vi "BonOMM-SAOMM.Test.vi"() -> ()   [LabVIEW 2011] (continued)
                        n5497 = property on="ModifRotation" class="Bool (strict)"("Blinking"=w3909) -> ()  [unwired: 2 in, 2 out]
                        n5498 = property on="ModifDome" class="Bool (strict)"("Blinking"=w3909) -> ()  [unwired: 2 in, 2 out]
                        n5499 = property on="Zénith" class="Bool (strict)"("Blinking"=w3909) -> ()  [unwired: 2 in, 2 out]
                        n5500 = property on="Range" class="Bool (strict)"("Blinking"=w3909) -> ()  [unwired: 2 in, 2 out]
                        n5501 = property on="Écran" class="Bool (strict)"("Blinking"=w3909) -> ()  [unwired: 2 in, 2 out]
                        n5502 = property on="ModifFoyer" class="Bool (strict)"("Blinking"=w3909) -> ()  [unwired: 2 in, 2 out]
                      }
                      frame #1 {
                        n5503 = control-ref of="TCS actif"() -> (w3916:refnum<vi>)
                        n5504 = local read "TCS VRN"() -> (w3929:refnum<visa-resource-name>)
                        n5505 = call "EXCOM-CMD.vi"("VRN IN"=w3929, "Bool Refnum"=w3916, "Commande #"=13) -> ("VRN OUT"=w3930:refnum<visa-resource-name>, "OK Done"=w3932:bool, "Error OUT"=w3931:errorcluster)  [unwired: 10 in]
                        n5506 = call "EXCOM-28.vi"("VISA resource name"=w3930, "Error IN"=w3931, "Bool Refnum"=w3916) -> ("VISA resource name dup"=w3917:refnum<visa-resource-name>, "NORA"=w3926:dbl, "NODEC"=w3925:dbl, "Error OUT"=w3927:errorcluster)  [unwired: 11 in, 2 out]
                        n5507 = local read "NO epoch"() -> (w3924:dbl)
                        n5508 = local read "LST"() -> (w3922:dbl)
                        n5509 = local write "TCS Error"(w3927) -> ()
                        n5510 = local write "TCS VRN"(w3917) -> ()
                        n5511 = call "Object_properties.vi"("Target RA"=w3926, "Target DEC"=w3925, "Target Epoch"=w3924, "Sideral Time"=w3922) -> ("NO RA"=w3921:string, "NO DEC"=w3920:string, "NO Epoch"=w3923:dbl, "NO HA"=w3918:dbl, "NO AM"=w3919:dbl)  [unwired: 7 in]
                        n5512 = local write "NO epoch"(w3923) -> ()
                        n5513 = local write "N.O. Déc."(w3920) -> ()
                        n5514 = local write "N.O. A.D."(w3921) -> ()
                        n5515 = local write "NO AM"(w3919) -> ()
                        n5516 = local write "NO HA"(w3918) -> ()
                      }
                    }
                    n5517 = case shown="False" w3907 {
                      selector: w3907 -> [w3933 w3937]
                      frame False {
                        n5518 = local write "StopTel"(w3933) -> ()
                        n5519 = One Button Dialog(message="ATTENTION!!\nLa commande STOP a échoué.\nVérifiez TCS.", button name ("OK")="OK" ("nom du bouton (\"OK\")")) -> ()  [unwired: 1 out]
                      }
                      frame True {
                        n5520 = Not(x=w3937) -> (.not. x?=w3936:bool)
                        n5521 = local write "StopTel"(w3936) -> ()
                      }
                    }
                  }
                }
              }
              event "cancel-raf": Mouse Down {
                # "Pas certain que ça fasse quoique ce soit ?!?"
                n5522 = event-data() -> ()  [unwired: 1 in, 8 out]
                n5523 = case shown="True" "cancel-raf" {
                  frame False {
                  }
                  frame True {
                    n5524 = local write "cancel-raf"(FALSE) -> ()
                    n5525 = control-ref of="TERMINAL"() -> (w3940:refnum<vi>)
                    n5526 = control-ref of="Indicateur d'état"() -> (w3941:refnum<vi>)
                    n5527 = call "TERMINAL.vi"("Indicateur Refnum"=w3941, "Terminal Refnum"=w3940, "Indicateur d'état"="Annulation du déplacement de la roue à filtre") -> ()
                    "Annulation en cours" <- TRUE
                  }
                }
              }
            }
            n5528 = local read "Quit"() -> (w3870:bool)
          }
          "Stops" <- w955
          n5529 = while {
            tunnel: [w2656] -> w954
            stop <- w2656 stop-if-true
            w2673 = 1.0
            # "Ajouté une condition sur l'état de la communication ?"
            # "Boucle de synchronisation avec StarryNight"
            n5530 = local read "AnnéeRL"() -> (w2657:dbl)
            n5531 = global read "Globals.vi" "ScopeSim._Telescope"() -> (w2669:refnum<k7>)
            n5532 = call "Get_SN_Coords.vi"("Output EPOCH"=w2657, "ScopeSim._Telescope"=w2669) -> ("DEC(sec)"=w2667:dbl, "RA(sec)"=w2668:dbl)  [unwired: 8 in]
            n5533 = local read "Dectmp"() -> (w2676:dbl)
            n5534 = local read "RAtmp"() -> (w2675:dbl)
            n5535 = Subtract(x=w2668, y=w2675) -> (x-y=w2674:dbl)
            n5536 = Subtract(x=w2676, y=w2667) -> (x-y=w2672:dbl)
            n5537 = Absolute Value(x=w2672) -> (abs(x)=w2670:dbl)
            n5538 = Absolute Value(x=w2674) -> (abs(x)=w2671:dbl)
            n5539 = Greater?(x=w2671, y=w2673) -> (0:w2666:bool)
            n5540 = Less Or Equal?(x=w2673, y=w2670) -> (x <= y?=w2663:bool)
            n5541 = Not Equal To 0?(x=w2668) -> (x != 0?=w2665:bool)
            n5542 = Not Equal To 0?(x=w2667) -> (x != 0?=w2662:bool)
            n5543 = And(x=w2665, y=w2666) -> (x .and. y?=w2664:bool)
            n5544 = And(x=w2663, y=w2662) -> (x .and. y?=w2661:bool)
            n5545 = Or(x=w2664, y=w2661) -> (x .or. y?=w2660:bool)
            n5546 = And(x="Sync_Ready", y=w2660) -> (x .and. y?=w2659:bool)
            n5547 = case shown="True" w2659 {
              tunnel: w2668 -> [_ w2691]
              tunnel: w2667 -> [_ w2693]
              tunnel: "Sync_Ready" -> [_ _]
              tunnel: w2657 -> [_ w2688]
              frame False {
                n5548 = global read "Globals.vi" "ScopeSim._Telescope"() -> (w2683:refnum<k7>)
                n5549 = local read "Epoch Tel"() -> (w2682:dbl)
                n5550 = local read "RA Tel"() -> (w2680:dbl)
                n5551 = local read "DEC Tel"() -> (w2681:dbl)
                n5552 = call "Set_SN_Coords.vi"("Coords EPOCH"=w2682, "input_DEC"=w2681, "input_RA"=w2680, "ScopeSim._Telescope"=w2683) -> ("precessed_DEC"=w2678:dbl, "precessed_RA"=w2679:dbl)  [unwired: 6 in]
                n5553 = local write "Dectmp"(w2678) -> ()
                n5554 = local write "RAtmp"(w2679) -> ()
              }
              frame True {
                # "Affiche les coordonnées dans l'époque\nd'affichage du télescope pour que la\ncomparaison soit facile."
                # "Mode test en attendant ..."
                n5555 = local read "Epoch Tel"() -> (w2689:dbl)
                n5556 = local write "RAtmp"(w2691) -> ()
                n5557 = local read "LST"() -> (w2692:dbl)
                n5558 = local write "Dectmp"(w2693) -> ()
                n5559 = call "Object_properties.vi"("Target RA"=w2691, "Target DEC"=w2693, "Target Epoch"=w2689, "Sideral Time"=w2692) -> ("NO RA"=w2685:string, "NO DEC"=w2684:string, "NO Epoch"=w2690:dbl, "NO HA"=w2686:dbl, "NO AM"=w2687:dbl)  [unwired: 7 in]
                n5560 = call "Mode sync(pop-up).vi"("Époq. in"=w2690, "Déc. in"=w2684, "RA in"=w2685) -> ("Valeur"=w2694:u32)
                n5561 = case shown="2" w2694 {
                  tunnel: w2691 -> [w2706 _ w2738 w2759]
                  tunnel: w2693 -> [w2705 _ w2739 w2758]
                  tunnel: w2689 -> [_ _ w2730 _]
                  tunnel: w2688 -> [_ _ w2729 w2755]
                  tunnel: w2687 -> [_ _ _ w2756]
                  tunnel: w2686 -> [_ _ _ w2757]
                  tunnel: w2685 -> [_ _ _ w2754]
                  tunnel: w2684 -> [_ _ _ w2753]
                  frame 0, Default {
                    w2695 = u16 1 items=["Region d'intérêt", "Prévisualisation"] ("ImageUsage")
                    # "Vérifier si ça marche ..."
                    n5562 = local read "AnnéeRL"() -> (w2702:dbl)
                    n5563 = local read "Epoch Tel"() -> (w2701:dbl)
                    n5564 = call "ad2deg.vi"("DEC (sec)"=w2705, "RA (sec)"=w2706) -> ("DEC (°)"=w2707:dbl, "RA (°)"=w2708:dbl)
                    n5565 = call "precess.vi"("Eq2"=w2701, "Eq1"=w2702, "DEC 1"=w2707, "RA 1"=w2708) -> ("DEC 2"=w2704:dbl, "RA 2"=w2703:dbl)
                    n5566 = global write "Globals.vi" "RA Tmp"(w2703) -> ()
                    n5567 = global write "Globals.vi" "DEC Tmp"(w2704) -> ()
                    n5568 = local read "ImgAstrom"() -> (w2716:T4)
                    n5569 = local read "FieldAstrom"() -> (w2719:T4)
                    n5570 = call "ad2xy.vi"("DEC"=w2704, "RA"=w2703, "Astrometry"=w2719) -> ("Y"=w2717:dbl, "X"=w2718:dbl)  [unwired: 6 in, 1 out]
                    n5571 = call "ad2xy.vi"("DEC"=w2704, "RA"=w2703, "Astrometry"=w2716) -> ("Y"=w2713:dbl, "X"=w2714:dbl)  [unwired: 6 in, 1 out]
                    n5572 = To Long Integer(number=w2714) -> (32bit integer=w2712:i32)
                    n5573 = To Long Integer(number=w2713) -> (32bit integer=w2711:i32)
                    n5574 = local read "ImgData"() -> (w2715:sgl[][])
                    n5575 = property on="TableXYPos" class="XYGraph (strict)"("Active Cursor"=u32 0, "Cursor.Cursor X"=w2718, "Cursor.Cursor Y"=w2717) -> ()  [unwired: 2 in, 2 out]
                    n5576 = call "subimage.vi"("Ysz/2"=100, "Xsz/2"=100, "Yc"=w2711, "Xc"=w2712, "ImgData"=w2715) -> ("SubImg"=w2699:sgl[][])  [unwired: 6 in]
                    n5577 = local write "SubIMG4DSS?"(TRUE ("SubIMG4DSS?")) -> ()
                    n5578 = Array Max & Min(array=w2699) -> (max value=w2700:sgl)  [unwired: 3 out]
                    n5579 = call "Draw_crosshair.vi"("Image IN"=w2699, "White Value"=w2700) -> ("Image OUT"=w2698:sgl[][])  [unwired: 13 in]
                    n5580 = local write "ImageUsage"(w2695) -> ()
                    n5581 = local write "subimg"(w2698) -> ()
                  }
                  frame 1 {
                    # "Annuler ..."
                    n5582 = control-ref of="TCS actif"() -> (w2720:refnum<vi>)
                    n5583 = local read "TCS VRN"() -> (w2721:refnum<visa-resource-name>)
                    n5584 = call "EXCOM-CMD.vi"("VRN IN"=w2721, "Bool Refnum"=w2720, "Commande #"=13) -> ("VRN OUT"=w2723:refnum<visa-resource-name>, "Error OUT"=w2724:errorcluster)  [unwired: 10 in, 1 out]
                    n5585 = local write "TCS Error"(w2724) -> ()
                    n5586 = local write "TCS VRN"(w2723) -> ()
                  }
                  frame 2 {
                    w2725 = u16 1 items=["Region d'intérêt", "Prévisualisation"] ("ImageUsage")
                    # "Les variables globales servent\npour l'éxécution de starast.vi\n(reste à confirmer l'époque)"
                    # "Devrait probablement vérifier la disponibilité de l'image d'abord."
                    # "Synchroniser la Cible"
                    n5587 = call "ad2deg.vi"("DEC (sec)"=w2739, "RA (sec)"=w2738) -> ("DEC (°)"=w2731:dbl, "RA (°)"=w2732:dbl)
                    n5588 = global write "Globals.vi" "RA Tmp"(w2738) -> ()
                    n5589 = global write "Globals.vi" "DEC Tmp"(w2739) -> ()
                    n5590 = call "precess.vi"("Eq2"=w2730, "Eq1"=w2729, "DEC 1"=w2731, "RA 1"=w2732) -> ("DEC 2"=w2727:dbl, "RA 2"=w2728:dbl)
                    n5591 = local read "ImgAstrom"() -> (w2750:T4)
                    n5592 = local read "FieldAstrom"() -> (w2751:T4)
                    n5593 = call "ad2xy.vi"("DEC"=w2727, "RA"=w2728, "Astrometry"=w2750) -> ("Y"=w2747:dbl, "X"=w2748:dbl)  [unwired: 6 in, 1 out]
                    n5594 = call "ad2xy.vi"("DEC"=w2727, "RA"=w2728, "Astrometry"=w2751) -> ("Y"=w2733:dbl, "X"=w2734:dbl)  [unwired: 6 in, 1 out]
                    n5595 = To Long Integer(number=w2748) -> (32bit integer=w2746:i32)
                    n5596 = To Long Integer(number=w2747) -> (32bit integer=w2745:i32)
                    n5597 = local read "ImgData"() -> (w2749:sgl[][])
                    n5598 = property on="TableXYPos" class="XYGraph (strict)"("Active Cursor"=u32 0, "Cursor.Cursor Position:Cursor X"=w2734, "Cursor.Cursor Position:Cursor Y"=w2733) -> ()  [unwired: 2 in, 2 out]
                    n5599 = call "subimage.vi"("Ysz/2"=100, "Xsz/2"=100, "Yc"=w2745, "Xc"=w2746, "ImgData"=w2749) -> ("SubImg"=w2741:sgl[][])  [unwired: 6 in]
                    n5600 = call "format_arcmin2arcsecstr.vi"("RA arcmin"=w2734, "DEC Arcmin"=w2733) -> ("Formatted RA"=w2737:string, "Formatted Dist"=w2735:string, "Formatted DEC"=w2736:string)  [unwired: 11 in]
                    n5601 = Array Max & Min(array=w2741) -> (max value=w2742:sgl)  [unwired: 3 out]
                    n5602 = call "Draw_crosshair.vi"("Image IN"=w2741, "White Value"=w2742) -> ("Image OUT"=w2740:sgl[][])  [unwired: 13 in]
                    n5603 = local write "SubIMG4DSS?"(TRUE ("SubIMG4DSS?")) -> ()
                    n5604 = local write "Cen-Cib-TOT"(w2735) -> ()
                    n5605 = local write "Cen-Cib-RA"(w2737) -> ()
                    n5606 = local write "Cen-Cib-DEC"(w2736) -> ()
                    n5607 = local write "ImageUsage"(w2725) -> ()
                    n5608 = local write "subimg"(w2740) -> ()
                  }
                  frame 4 {
                    # "À confirmer ..."
                    # "On envoie toujours les coordonnées en JNOW puisque Starry Night\nn'est pas capable de précesser des coordonnées correctement."
                    # "Synchroniser les coordonnées du télescope"
                    n5609 = local write "NO epoch"(w2755) -> ()
                    n5610 = expression code="x/3600."(w2758) -> (w2766:dbl)
                    n5611 = local write "N.O. A.D."(w2754) -> ()
                    n5612 = local write "N.O. Déc."(w2753) -> ()
                    n5613 = expression code="x/3600."(w2759) -> (w2765:dbl)
                    n5614 = Build Array(w2765, w2766, w2755) -> (w2767:dbl[])
                    n5615 = control-ref of="TCS actif"() -> (w2760:refnum<vi>)
                    n5616 = local read "TCS VRN"() -> (w2761:refnum<visa-resource-name>)
                    n5617 = call "EXCOM-CMD.vi"("VRN IN"=w2761, "Bool Refnum"=w2760, "Commande #"=6, "Args"=w2767) -> ("VRN OUT"=w2764:refnum<visa-resource-name>, "Error OUT"=w2763:errorcluster)  [unwired: 9 in, 1 out]
                    n5618 = local write "TCS Error"(w2763) -> ()
                    n5619 = local write "TCS VRN"(w2764) -> ()
                    "NO HA" <- w2757
                    "NO AM" <- w2756
                  }
                }
              }
            }
            n5620 = Wait Until Next ms Multiple(millisecond multiple=u32 500) -> ()  [unwired: 1 out]
            n5621 = local read "Quit"() -> (w2656:bool)
          }
          "Synchro StarryNight" <- w954
        }
      }
      n5622 = local write "QuitInitialization"(TRUE ("QuitInitialization")) -> ()
    }
    frame #9 {
      # "Cloture"
      n5623 = global read "Globals.vi" "BonOMM VI Refnum"() -> (w7395:refnum<vi>)
      n5624 = stacked-sequence {
        tunnel: w7395 -> [w7401 _ _ w7460 _ _]
        tunnel: w7396 -> [_ w7429 _ _ _ _]
        frame #0 {
          w7402 = FALSE
          w7427 = bool[] [FALSE, FALSE, FALSE]  # Array Constant
          # "Gestion dans le menu à revoir ..."
          n5625 = property class="VI"(reference=w7401) -> ("Front Panel.PanelBounds"=→"Front Panel Window:Panel Bounds":T6, "Minimum Panel Size"=→"Front Panel Window:Minimum Size":T5)  [unwired: 1 in, 2 out]
          n5626 = property on="Pane" class="Pane"() -> ("Origin"=→"Origin":T5)  [unwired: 2 in, 2 out]
          n5627 = Current VI's Menubar() -> (w7409:refnum<k9>)
          n5628 = Get Menu Item Info(7:"Affichage" ("item tag"), 11:w7409) -> (5:w7408:string[])  [unwired: 1 in, 6 out]
          n5629 = local write "Status lamp"(w7427) -> ()
          n5630 = Index Array(array=w7408, index #1=0 ("indice"), index #2=1 ("indice"), index #3=2 ("indice"), index #4=3 ("indice"), index #5=4 ("indice"), index #6=7 ("indice")) -> (element #1=w7420:string, element #2=w7419:string, element #3=w7418:string, element #4=w7417:string, element #5=w7416:string, element #6=w7404:string)
          n5631 = local read "Calib VRN"() -> (w7426:refnum<visa-resource-name>)
          n5632 = Current VI's Menubar() -> (w7405:refnum<k9>)
          n5633 = call "Controle_des_lampe.vi"("VISA resource name"=w7426, "Status In"=w7427) -> ()  [unwired: 3 out]
          n5634 = Get Menu Item Info(7:w7420, 11:w7405) -> (4:w7425:bool)  [unwired: 1 in, 6 out]
          n5635 = Get Menu Item Info(7:w7419, 11:w7405) -> (4:w7424:bool)  [unwired: 1 in, 6 out]
          n5636 = Get Menu Item Info(7:w7418, 11:w7405) -> (4:w7423:bool)  [unwired: 1 in, 6 out]
          n5637 = Get Menu Item Info(7:w7417, 11:w7405) -> (4:w7422:bool)  [unwired: 1 in, 6 out]
          n5638 = Get Menu Item Info(7:w7416, 11:w7405) -> (4:w7421:bool)  [unwired: 1 in, 6 out]
          n5639 = Get Menu Item Info(7:w7404, 11:w7405) -> (4:w7403:bool)  [unwired: 1 in, 6 out]
          n5640 = Build Array(w7425, w7424, w7423, w7422, w7421, w7402, w7402, w7403) -> (→"Éléments cochés":bool[])
        }
        frame #1 {
          n5641 = case shown="True" w7429 {
            frame False {
            }
            frame True {
              n5642 = local read "Table VRN"() -> (w7439:refnum<visa-resource-name>)
              n5643 = VISA Close(VISA resource name=w7439) -> (error out=w7434:errorcluster)  [unwired: 1 in]
              n5644 = local write "Table Error"(w7434) -> ()
              n5645 = global read "Globals.vi" "CameraTuning VI Refnum"() -> (w7437:refnum<vi>)
              n5646 = local read "TCS VRN"() -> (w7443:refnum<visa-resource-name>)
              n5647 = global read "Globals.vi" "ScopeSim._Telescope"() -> (w7438:refnum<k7>)
              n5648 = VISA Close(VISA resource name=w7443) -> (error out=w7433:errorcluster)  [unwired: 1 in]
              n5649 = local read "PrAMS VRN"() -> (w7442:refnum<visa-resource-name>)
              n5650 = Close Reference(reference=w7438) -> (error out=w7435:errorcluster)  [unwired: 1 in]
              n5651 = Close Reference(reference=w7437) -> (error out=w7436:errorcluster)  [unwired: 1 in]
              n5652 = local write "Starry Night Error"(w7435) -> ()
              n5653 = local write "VI Reference Error"(w7436) -> ()
              n5654 = VISA Close(VISA resource name=w7442, error in (no error)=w7433) -> (error out=w7432:errorcluster)
              n5655 = local read "Excmd VRN"() -> (w7441:refnum<visa-resource-name>)
              n5656 = local write "TCS Error"(w7432) -> ()
              n5657 = VISA Close(VISA resource name=w7441) -> (error out=w7431:errorcluster)  [unwired: 1 in]
              n5658 = local read "Calib VRN"() -> (w7440:refnum<visa-resource-name>)
              n5659 = local write "Excom Error"(w7431) -> ()
              n5660 = VISA Close(VISA resource name=w7440) -> (error out=w7430:errorcluster)  [unwired: 1 in]
              n5661 = local write "Serial Error"(w7430) -> ()
            }
          }
          n5662 = global read "Global.vi" "events"() -> (w7428:refnum<queue>)
          n5663 = Flush Queue(queue=w7428) -> ()  [unwired: 1 in, 3 out]
        }
        frame #2 {
          # "Remplacer par un VI qui gère la déconnexion de PrAMS et Hexapode-Console"
          n5664 = disable-structure shown="Disabled" {
            frame Disabled {
              n5665 = local read "MessageType"() -> (w7446:cluster{string[], u32[]})
              n5666 = control-ref of="PrAMS actif"() -> (w7450:refnum<vi>)
              n5667 = control-ref of="PrAMS-ACK"() -> (w7449:refnum<vi>)
              n5668 = local read "PrAMS Error"() -> (w7447:errorcluster)
              n5669 = local read "PrAMS VRN"() -> (w7451:refnum<visa-resource-name>)
              n5670 = local read "Signature"() -> (w7448:u32)
              n5671 = call "SAOMM-SendSET.vi"("PRAMMS-COMM IN"=w7451, "Active Refnum"=w7450, "PrAMS-ACK"=w7449, "Signature"=w7448, "Error IN"=w7447, "MessageType"=w7446, "Active SET"="emtStopAcquisition", "Value (little endianed byte array)"=u8[] []) -> ()  [unwired: 4 in, 4 out]
            }
            frame Enabled {
            }
          }
        }
        frame #3 {
          # "Enregistrement de l'état des contrôles et indicateurs\ndans les fichiers controls.data et indicators.data"
          n5672 = local read "path_config"() -> (w7453:path)
          n5673 = invoke class="VI" method="Ctrl Val.Get All"(reference=w7460, "Controls"=TRUE ("controls")) -> (reference out=w7477:refnum<vi>, error out=w7471:errorcluster, "Get All Control Values Variant"=w7459:cluster{"Name":string, "Variant Data":variant}[])  [unwired: 2 in, 1 out]
          n5674 = Build Path(base path=w7453, name or relative path="controls.data") -> (appended path=w7466:path)
          n5675 = Delete(path (use dialog)=w7466) -> (deleted path=w7465:path)  [unwired: 4 in, 2 out]
          n5676 = Flatten To String(anything=w7459) -> (data string=w7470:string)  [unwired: 3 in, 2 out]
          n5677 = for {
            tunnel: w7459 -> [w7479] mode=indexing
            tunnel: [w7478] -> w7458 mode=indexing
            n5678 = Unbundle(w7479) -> ("Name"=w7478:string)  [unwired: 1 out]
          }
          n5679 = call "Write Characters To File (no popup).vi"("append to file? (new file:F)"=FALSE, "character string"=w7470, "file path (dialog if empty)"=w7465) -> ()  [unwired: 2 in, 1 out]
          n5680 = local read "CtrlName"() -> (w7457:string[])
          n5681 = Not Equal?(x=w7457, y=w7458) -> (x != y?=w7456:bool[])
          n5682 = Boolean Array To Number(Boolean array=w7456) -> (number=w7455:u32)
          n5683 = invoke class="VI" method="Ctrl Val.Get All"(reference=w7477, error in=w7471, "Controls"=FALSE ("controls")) -> (reference out=w7462:refnum<vi>, error out=w7461:errorcluster, "Get All Control Values Variant"=w7472:cluster{"Name":string, "Variant Data":variant}[])  [unwired: 1 in, 1 out]
          n5684 = Greater Than 0?(x=w7455) -> (x > 0?=w7454:bool)
          n5685 = local write "CtrlGetErrInd"(w7454) -> ()
          n5686 = Build Path(base path=w7453, name or relative path="indicators.data") -> (appended path=w7464:path)
          n5687 = Delete(path (use dialog)=w7464) -> (deleted path=w7463:path)  [unwired: 4 in, 2 out]
          n5688 = Flatten To String(anything=w7472) -> (data string=w7469:string)  [unwired: 3 in, 2 out]
          n5689 = call "Write Characters To File (no popup).vi"("append to file? (new file:F)"=FALSE, "character string"=w7469, "file path (dialog if empty)"=w7463) -> ()  [unwired: 2 in, 1 out]
          n5690 = Close Reference(reference=w7462, error in (no error)=w7461) -> (error out=w7452:errorcluster)
          n5691 = local write "Config Error"(w7452) -> ()
        }
        frame #4 {
          w7489 = "LVDTs" ("key")
          w7497 = i16 3 ("precision (6)")
          w7498 = T63."exponential" ("format (fractional)")
          w7504 = "tables"
          w7499 = "variables"
          # "Enregistrement dans le fichier \"properties.ini\""
          n5692 = local read "properties.ini"() -> (w7521:path)
          n5693 = call <vilib>:"Open Config Data.vi"("create file if necessary (T)"=FALSE, "configuration file path"=w7521) -> ("error out"=w7522:errorcluster, "refnum"=w7523:T24)  [unwired: 7 in, 1 out]
          n5694 = local read "k0_focus"() -> (w7555:dbl)
          n5695 = call-poly <vilib>:"Write Key.vi"("section"=w7499, "error in (no error)"=w7522, "value"=w7555, "key"="k0_focus", "refnum"=w7523) -> ("error out"=w7549:errorcluster, "refnum out"=w7553:T24)  [unwired: 4 in, 1 out]
          n5696 = local read "k1_focus"() -> (w7545:dbl)
          n5697 = call-poly <vilib>:"Write Key.vi"("section"=w7499, "error in (no error)"=w7549, "value"=w7545, "key"="k1_focus", "refnum"=w7553) -> ("error out"=w7548:errorcluster, "refnum out"=w7552:T24)  [unwired: 4 in, 1 out]
          n5698 = local read "a1_focus"() -> (w7543:dbl)
          n5699 = call-poly <vilib>:"Write Key.vi"("format (fractional)"=w7498, "precision (6)"=w7497, "section"=w7499, "error in (no error)"=w7548, "value"=w7543, "key"="a1_focus", "refnum"=w7552) -> ("error out"=w7547:errorcluster, "refnum out"=w7551:T24)  [unwired: 2 in, 1 out]
          n5700 = local read "a2_focus"() -> (w7540:dbl)
          n5701 = call-poly <vilib>:"Write Key.vi"("format (fractional)"=w7498, "precision (6)"=w7497, "section"=w7499, "error in (no error)"=w7547, "value"=w7540, "key"="a2_focus", "refnum"=w7551) -> ("error out"=w7546:errorcluster, "refnum out"=w7550:T24)  [unwired: 2 in, 1 out]
          n5702 = local read "a3_focus"() -> (w7538:dbl)
          n5703 = call-poly <vilib>:"Write Key.vi"("format (fractional)"=w7498, "precision (6)"=w7497, "section"=w7499, "error in (no error)"=w7546, "value"=w7538, "key"="a3_focus", "refnum"=w7550) -> ("error out"=w7480:errorcluster, "refnum out"=w7481:T24)  [unwired: 2 in, 1 out]
          n5704 = local read "dflt-EQX"() -> (w7500:dbl)
          n5705 = call-poly <vilib>:"Write Key.vi"("section"=w7499, "error in (no error)"=w7480, "value"=w7500, "key"="equinox", "refnum"=w7481) -> ("error out"=w7492:errorcluster, "refnum out"=w7496:T24)  [unwired: 4 in, 1 out]
          n5706 = local read "LVDT-zero"() -> (w7482:dbl)
          n5707 = call-poly <vilib>:"Write Key.vi"("section"=w7489, "error in (no error)"=w7492, "value"=w7482, "key"="ra-zero", "refnum"=w7496) -> ("error out"=w7491:errorcluster, "refnum out"=w7495:T24)  [unwired: 4 in, 1 out]
          n5708 = local read "LVDT-scale"() -> (w7484:dbl)
          n5709 = call-poly <vilib>:"Write Key.vi"("section"=w7489, "error in (no error)"=w7491, "value"=w7484, "key"="ra-scale", "refnum"=w7495) -> ("error out"=w7490:errorcluster, "refnum out"=w7494:T24)  [unwired: 4 in, 1 out]
          n5710 = local read "LVDT-time"() -> (w7483:dbl)
          n5711 = call-poly <vilib>:"Write Key.vi"("section"=w7489, "error in (no error)"=w7490, "value"=w7483, "key"="acq-time", "refnum"=w7494) -> ("error out"=w7485:errorcluster, "refnum out"=w7493:T24)  [unwired: 4 in, 1 out]
          n5712 = local read "vitesse rapide"() -> (w7515:dbl)
          n5713 = call-poly <vilib>:"Write Key.vi"("section"=w7504, "error in (no error)"=w7485, "value"=w7515, "key"="vrapid", "refnum"=w7493) -> ("error out"=w7508:errorcluster, "refnum out"=w7510:T24)  [unwired: 4 in, 1 out]
          n5714 = local read "vitesse lente"() -> (w7516:dbl)
          n5715 = call-poly <vilib>:"Write Key.vi"("section"=w7504, "error in (no error)"=w7508, "value"=w7516, "key"="vlente", "refnum"=w7510) -> ("error out"=w7507:errorcluster, "refnum out"=w7509:T24)  [unwired: 4 in, 1 out]
          n5716 = local read "accelleration"() -> (w7517:dbl)
          n5717 = call-poly <vilib>:"Write Key.vi"("section"=w7504, "error in (no error)"=w7507, "value"=w7517, "key"="accel", "refnum"=w7509) -> ("error out"=w7518:errorcluster, "refnum out"=w7519:T24)  [unwired: 4 in, 1 out]
          n5718 = local read "vitesse focus"() -> (w7520:dbl)
          n5719 = call-poly <vilib>:"Write Key.vi"("section"=w7504, "error in (no error)"=w7518, "value"=w7520, "key"="vfocus", "refnum"=w7519) -> ("error out"=w7505:errorcluster, "refnum out"=w7506:T24)  [unwired: 4 in, 1 out]
          n5720 = local read "CentreTel X"() -> (w7529:dbl)
          n5721 = call-poly <vilib>:"Write Key.vi"("section"=w7504, "error in (no error)"=w7505, "value"=w7529, "key"="cenx", "refnum"=w7506) -> ("error out"=w7536:errorcluster, "refnum out"=w7534:T24)  [unwired: 4 in, 1 out]
          n5722 = local read "CentreTel Y"() -> (w7528:dbl)
          n5723 = call-poly <vilib>:"Write Key.vi"("section"=w7504, "error in (no error)"=w7536, "value"=w7528, "key"="ceny", "refnum"=w7534) -> ("error out"=w7537:errorcluster, "refnum out"=w7535:T24)  [unwired: 4 in, 1 out]
          n5724 = local read "Reference X"() -> (w7527:dbl)
          n5725 = call-poly <vilib>:"Write Key.vi"("section"=w7504, "error in (no error)"=w7537, "value"=w7527, "key"="refX", "refnum"=w7535) -> ("error out"=w7526:errorcluster, "refnum out"=w7525:T24)  [unwired: 4 in, 1 out]
          n5726 = local read "Reference Y"() -> (w7524:dbl)
          n5727 = call-poly <vilib>:"Write Key.vi"("section"=w7504, "error in (no error)"=w7526, "value"=w7524, "key"="refY", "refnum"=w7525) -> ("error out"=w7502:errorcluster, "refnum out"=w7503:T24)  [unwired: 4 in, 1 out]
          n5728 = call <vilib>:"Close Config Data.vi"("error in (no error)"=w7502, "refnum"=w7503) -> ()  [unwired: 8 in, 2 out]
        }
        frame #5 {
          n5729 = call "Enregistrement des parametres.vi"() -> ()  [unwired: 1 in]
        }
      }
      n5730 = case shown="True" w7394 {
        selector: w7394 -> [_ w7397]
        frame False {
        }
        frame True {
          n5731 = property on="filtre_nom" class="Str"("Visible"=w7397) -> ()  [unwired: 2 in, 2 out]
          n5732 = property on="q-raf" class="Bool (strict)"("Visible"=w7397) -> ()  [unwired: 2 in, 2 out]
          n5733 = property on="cancel-raf" class="Bool (strict)"("Visible"=w7397) -> ()  [unwired: 2 in, 2 out]
          n5734 = property on="change_filtre_liste" class="Bool (strict)"("Visible"=w7397) -> ()  [unwired: 2 in, 2 out]
          n5735 = property on="StopCam" class="Bool (strict)"("Visible"=w7397) -> ()  [unwired: 2 in, 2 out]
          n5736 = property on="GoCam" class="Bool (strict)"("Visible"=w7397) -> ()  [unwired: 2 in, 2 out]
          n5737 = property on="F#" class="DigNum (strict)"("Visible"=w7397) -> ()  [unwired: 2 in, 2 out]
          n5738 = property on="ChoixFiltre" class="Clust (strict)"("Visible"=w7397) -> ()  [unwired: 2 in, 2 out]
          n5739 = property on="ST_RAZ" class="Bool"("Visible"=w7397) -> ()  [unwired: 2 in, 2 out]
          n5740 = property on="ST-" class="Bool (strict)"("Visible"=w7397) -> ()  [unwired: 2 in, 2 out]
          n5741 = property on="ST+" class="Bool (strict)"("Visible"=w7397) -> ()  [unwired: 2 in, 2 out]
          n5742 = property on="SET ZERO" class="Bool"("Visible"=w7397) -> ()  [unwired: 2 in, 2 out]
        }
      }
      n5743 = property on="Approaching limit" class="Bool (strict)"("Visible"=w7394, "Blinking"=w7394) -> ()  [unwired: 2 in, 2 out]
      n5744 = property on="Target OutofRange" class="Bool (strict)"("Visible"=w7394, "Blinking"=w7394) -> ()  [unwired: 2 in, 2 out]
    }
  }
  n5745 = while {
    stop <- w7564 stop-if-true
    w7566 = T64 {"message"="", "data"=variant}  # event
    n5746 = Obtain Queue(element data type=w7566) -> (queue out=w7565:refnum<queue>)  [unwired: 4 in, 2 out]
    n5747 = global write "Global.vi" "events"(w7565) -> ()
    n5748 = Dequeue Element(queue=w7565) -> (queue out=w7562:refnum<queue>, element=w7563:T64, error out=w7564:errorcluster)  [unwired: 2 in, 1 out]
    n5749 = Unbundle By Name(w7563) -> ("message"=w7560:string, "data"=w7561:variant)
    n5750 = Match Pattern(string=w7560, regular expression="[.]") -> (before substring=w7559:string, after substring=w7557:string)  [unwired: 1 in, 2 out]
    n5751 = case shown="\"Foyer\"" w7559 {
      tunnel: w7562 -> [_ _]
      tunnel: w7561 -> [_ w7567]
      tunnel: w7557 -> [_ w7568]
      frame "False", Default {
      }
      frame "Foyer" {
        n5752 = case shown="\"Ajuster\"" w7568 {
          tunnel: w7567 -> [_ w7574 w7684]
          frame "False", Default {
          }
          frame "Ajuster" {
            n5753 = Variant To Data(type=T22 {"newFoyer"=0.0, "updSonde"=TRUE, "oldFoyer"=0.0}, Variant=w7574) -> (data=w7573:T22)  [unwired: 1 in, 1 out]
            n5754 = Unbundle By Name(w7573) -> ("newFoyer"=w7571:dbl, "updSonde"=w7570:bool, "oldFoyer"=w7569:dbl)
            n5755 = stacked-sequence {
              tunnel: w7571 -> [_ w7583 _]
              tunnel: w7570 -> [_ w7584 _]
              tunnel: w7569 -> [_ w7582 _]
              frame #0 {
                w7579 = 2
                n5756 = control-ref of="TERMINAL"() -> (w7577:refnum<vi>)
                n5757 = control-ref of="Indicateur d'état"() -> (w7576:refnum<vi>)
                n5758 = call "TERMINAL.vi"("Indicateur Refnum"=w7576, "Terminal Refnum"=w7577, "Indicateur d'état"="Modification logicielle du foyer") -> ()
                n5759 = property on="ModCoor" class="Bool (strict)"("Disabled"=w7579) -> ()  [unwired: 2 in, 2 out]
                n5760 = property on="Synctel" class="Bool (strict)"("Disabled"=w7579) -> ()  [unwired: 2 in, 2 out]
                n5761 = property on="Offset OK" class="Bool (strict)"("Disabled"=w7579) -> ()  [unwired: 2 in, 2 out]
                n5762 = property on="Zénith" class="Bool (strict)"("Disabled"=w7579) -> ()  [unwired: 2 in, 2 out]
                n5763 = property on="GO" class="Bool (strict)"("Disabled"=w7579) -> ()  [unwired: 2 in, 2 out]
                n5764 = property on="ModifFoyer" class="Bool (strict)"("Blinking"=TRUE) -> ()  [unwired: 2 in, 2 out]
                n5765 = property on="ModifRotation" class="Bool (strict)"("Disabled"=w7579) -> ()  [unwired: 2 in, 2 out]
                n5766 = property on="Range" class="Bool (strict)"("Disabled"=w7579) -> ()  [unwired: 2 in, 2 out]
                n5767 = property on="ModifDome" class="Bool (strict)"("Disabled"=w7579) -> ()  [unwired: 2 in, 2 out]
                n5768 = property on="Coupole-Tél" class="Bool (strict)"("Disabled"=w7579) -> ()  [unwired: 2 in, 2 out]
                n5769 = property on="Écran" class="Bool (strict)"("Disabled"=w7579) -> ()  [unwired: 2 in, 2 out]
              }
              frame #1 {
                n5770 = control-ref of="TCS actif"() -> (w7581:refnum<vi>)
                n5771 = local read "TCS VRN"() -> (w7580:refnum<visa-resource-name>)
                n5772 = while {
                  tunnel: w7580 -> [w7607]
                  tunnel: w7584 -> [w7606]
                  tunnel: w7583 -> [w7605]
                  tunnel: w7582 -> [w7602]
                  tunnel: w7581 -> [w7593]
                  i -> [w7598]
                  stop <- w7599 stop-if-true
                  n5773 = Build Array(w7605) -> (w7590:dbl[])
                  n5774 = call "EXCOM-CMD.vi"("VRN IN"=w7607, "Bool Refnum"=w7593, "Commande #"=27 ("NombredArguments"), "Args"=w7590) -> ("VRN OUT"=w7589:refnum<visa-resource-name>, "OK Done"=w7592:bool, "Error OUT"=w7588:errorcluster)  [unwired: 9 in]
                  n5775 = case shown="True" w7592 {
                    tunnel: w7589 -> [w7609 w7621]
                    tunnel: w7606 -> [_ w7620]
                    tunnel: w7605 -> [_ w7619]
                    tunnel: [TRUE w7618] -> w7595
                    tunnel: w7588 -> [w7608 w7617]
                    tunnel: [w7609 w7616] -> w7587
                    tunnel: [w7608 w7615] -> w7586
                    tunnel: w7593 -> [_ w7614]
                    tunnel: [_ w7613] -> w7585
                    frame False {
                      n5776 = One Button Dialog(message="ATTENTION!!\nLa commande MODIF-FOYER a échoué.\nRecommencez ou vérifiez TCS.", button name ("OK")="OK" ("nom du bouton (\"OK\")")) -> ()  [unwired: 1 out]
                    }
                    frame True {
                      n5777 = stacked-sequence {
                        tunnel: w7621 -> [_ w7632 _ _]
                        tunnel: w7620 -> [_ _ w7675 _]
                        tunnel: w7619 -> [_ _ w7676 _]
                        tunnel: [_ w7631 _ _] -> w7618
                        tunnel: w7617 -> [_ w7630 _ _]
                        tunnel: [_ w7627 _ _] -> w7616
                        tunnel: [_ w7626 _ _] -> w7615
                        tunnel: w7614 -> [_ w7624 _ _]
                        tunnel: [_ _ _ w7679] -> w7613
                        frame #0 {
                          # "Encore une fois, on devrait vérifier avec les bits d'états ..."
                          # "attendre 1s que la commande soit acceptée par TCS"
                          n5778 = Wait (ms)(milliseconds to wait=u32 1000 ("attente (ms)")) -> ()  [unwired: 1 out]
                        }
                        frame #1 {
                          # "Changement de  la valeur du foyer."
                          n5779 = Tick Count (ms)() -> (millisecond timer value=w7633:u32)
                          n5780 = while {
                            tunnel: w7633 -> [w7647]
                            tunnel: [w7644] -> w7631
                            tunnel: w7632 -> [w7639]
                            tunnel: w7630 -> [w7638]
                            tunnel: [w7637] -> w7629
                            tunnel: [w7636] -> w7628
                            tunnel: [w7635] -> w7625
                            tunnel: w7624 -> [w7634]
                            tunnel: [w7634] -> w7623
                            stop <- w7646 stop-if-true
                            n5781 = Tick Count (ms)() -> (millisecond timer value=w7648:u32)
                            n5782 = call "EXCOM-26.vi"("VRN IN"=w7639, "Bool Refnum"=w7634, "Error IN"=w7638) -> ("VRN OUT"=w7637:refnum<visa-resource-name>, "OK Done"=w7635:bool, "STATEX"=w7640:bool[], "Error OUT"=w7636:errorcluster)  [unwired: 6 in, 3 out]
                            n5783 = Subtract(x=w7648, y=w7647) -> (x-y=w7649:u32)
                            n5784 = Greater?(x=w7649, y=u32 180000) -> (0:w7644:bool)
                            n5785 = Index Array(array=w7640, index=0 ("Index")) -> (element=w7641:bool)
                            n5786 = Not(x=w7641) -> (.not. x?=w7643:bool)
                            n5787 = Or(x=w7643, y=w7644) -> (x .or. y?=w7646:bool)
                            n5788 = Wait Until Next ms Multiple(millisecond multiple=u32 500 ("n millisecondes")) -> ()  [unwired: 1 out]
                          }
                          n5789 = case shown="True" w7631 {
                            tunnel: w7629 -> [w7652 w7658]
                            tunnel: w7628 -> [w7651 w7657]
                            tunnel: [w7652 w7656] -> w7627
                            tunnel: [w7651 w7655] -> w7626
                            tunnel: w7625 -> [_ w7654]
                            tunnel: w7623 -> [_ w7653]
                            frame False {
                            }
                            frame True {
                              n5790 = One Button Dialog(message="ATTENTION!!\nProblème d'ajustement\ndu foyer du télescope.\nVérifiez TCS.", button name ("OK")="OK" ("nom du bouton (\"OK\")")) -> (true=w7660:bool)
                              n5791 = case shown="True" w7660 {
                                tunnel: w7658 -> [w7663 w7669]
                                tunnel: w7657 -> [w7662 w7668]
                                tunnel: [w7663 w7667] -> w7656
                                tunnel: [w7662 w7666] -> w7655
                                tunnel: w7654 -> [_ _]
                                tunnel: w7653 -> [_ w7664]
                                frame False {
                                }
                                frame True {
                                n5792 = call "EXCOM-CMD.vi"("VRN IN"=w7669, "Bool Refnum"=w7664, "Commande #"=13 ("NombredArguments"), "Error IN"=w7668) -> ("VRN OUT"=w7667:refnum<visa-resource-name>, "OK Done"=w7665:bool, "Error OUT"=w7666:errorcluster)  [unwired: 9 in]
                                n5793 = case shown="False" w7665 {
                                frame False {
                                n5794 = One Button Dialog(message="ATTENTION!!\nLa commande STOP a échoué.\nVérifiez TCS.", button name ("OK")="OK" ("nom du bouton (\"OK\")")) -> ()  [unwired: 1 out]
                                }
                                frame True {
                                n5795 = Wait (ms)(milliseconds to wait=u32 10 ("attente (ms)")) -> ()  [unwired: 1 out]
                                }
                                }
                                }
                              }
                            }
                          }
                        }
                        frame #2 {
                          n5796 = case shown="True" w7675 {
                            tunnel: w7676 -> [_ w7677]
                            frame False {
                            }
                            frame True {
                              n5797 = call "EnqueueEvents.vi"("data"=w7677, "message"="Foyer.Sonde") -> ()  [unwired: 1 in]
                            }
                          }
                          n5798 = Wait (ms)(milliseconds to wait=u32 750) -> ()  [unwired: 1 out]
                        }
                        frame #3 {
                          n5799 = local read "Foyer"() -> (w7679:dbl)
                        }
                      }
                    }
                  }
                  n5800 = local read "Annulation du foyer"() -> (w7594:bool)
                  n5801 = Subtract(x=w7585, y=w7602) -> (x-y=w7604:dbl)
                  n5802 = local write "TCS VRN"(w7587) -> ()
                  n5803 = Greater?(x=w7598, y=2) -> (0:w7596:bool)
                  n5804 = local write "TCS Error"(w7586) -> ()
                  n5805 = Absolute Value(x=w7604) -> (abs(x)=w7603:dbl)
                  n5806 = Greater?(x=w7603, y=1.0) -> (0:w7600:bool)
                  n5807 = Compound Arithmetic op=OR(w7600, w7596, w7595, w7594) -> (w7599:bool)
                }
              }
              frame #2 {
                w7681 = 0
                w7680 = FALSE
                n5808 = property on="ModifDome" class="Bool (strict)"("Disabled"=w7681) -> ()  [unwired: 2 in, 2 out]
                n5809 = property on="Écran" class="Bool (strict)"("Disabled"=w7681) -> ()  [unwired: 2 in, 2 out]
                n5810 = property on="Range" class="Bool (strict)"("Disabled"=w7681) -> ()  [unwired: 2 in, 2 out]
                n5811 = property on="Zénith" class="Bool (strict)"("Disabled"=w7681) -> ()  [unwired: 2 in, 2 out]
                n5812 = property on="Synctel" class="Bool (strict)"("Disabled"=w7681) -> ()  [unwired: 2 in, 2 out]
                n5813 = property on="Offset OK" class="Bool (strict)"("Disabled"=w7681) -> ()  [unwired: 2 in, 2 out]
                n5814 = property on="GO" class="Bool (strict)"("Disabled"=w7681) -> ()  [unwired: 2 in, 2 out]
                n5815 = property on="ModCoor" class="Bool (strict)"("Disabled"=w7681) -> ()  [unwired: 2 in, 2 out]
                n5816 = property on="ModifRotation" class="Bool (strict)"("Disabled"=w7681) -> ()  [unwired: 2 in, 2 out]
                n5817 = property on="Coupole-Tél" class="Bool (strict)"("Disabled"=w7681) -> ()  [unwired: 2 in, 2 out]
                n5818 = local write "Annulation du foyer"(w7680) -> ()
                n5819 = property on="ModifFoyer" class="Bool (strict)"("Blinking"=w7680) -> ()  [unwired: 2 in, 2 out]
                n5820 = local write "ModifFoyer"(w7680) -> ()
              }
            }
          }
          frame "Sonde" {
            n5821 = local read "Foyer"() -> (w7683:dbl)
            n5822 = Variant To Data(type=w7683, Variant=w7684) -> (data=w7682:dbl)  [unwired: 1 in, 1 out]
            n5823 = formula code="foyersonde=foyertel*k1+k0;"("foyertel"=w7682, "k0"="k0_focus", "k1"="k1_focus") -> ("foyersonde"=w7687:dbl)
            n5824 = local read "CentreTel X"() -> (w7694:dbl)
            n5825 = local read "CentreTel Y"() -> (w7693:dbl)
            n5826 = local read "Position X"() -> (w7686:dbl)
            n5827 = local read "Position Y"() -> (w7685:dbl)
            n5828 = local read "a1_focus"() -> (w7691:dbl)
            n5829 = local read "a2_focus"() -> (w7690:dbl)
            n5830 = local read "a3_focus"() -> (w7689:dbl)
            n5831 = call "Calc_focus.vi"("Pos X"=w7686, "Pos Y"=w7685, "Cen X"=w7694, "Cen Y"=w7693, "a1"=w7691, "a2"=w7690, "a3"=w7689) -> ("Residu"=w7692:dbl)  [unwired: 7 in, 1 out]
            n5832 = Subtract(x=w7687, y=w7692) -> (x-y=w7688:dbl)
            n5833 = local write "FoyerAuCentre"(w7688) -> ()
          }
        }
      }
    }
  }
